vi "S4ACS_GUI.vi"() -> ()   [LabVIEW 2012]
uses:
  StateMachine/State Machine.lvclass
  Interface/Interface.lvclass
  S4ACS_GUI/S4ACS_GUI.lvclass
  Channel/Channel.lvclass
  Acquisition/Acquisition.lvclass
  Trigger/Trigger.lvclass
  SyncBox/Sync Box.lvclass
panel:
  in  "SyncBox Setup":enum32{"Page 1"}(tab)
  in  "Set SyncBox":bool
  in  "DelayA":string
  in  "DelayB":string
  in  "DelayC":string
  in  "DelayD":string
  in  "SyncBox":bool
  in  "DS9":bool
  in  "Comments":string
  in  "Observation Title":string
  in  "Image Path":path
  in  "File Basename":string
  in  "# Index":u32
  in  "# Images":u32
  out "error out":errorcluster
  in  "Kinetic Series Length":u8=1 min=1 max=80
  in  "Final Line":u16=1024 min=1 max=1024
  in  "Image Name":string="CH1"
  in  "Final Column":u16=1024 min=1 max=1024
  in  "Initial Cloumn":u16=1 min=1 max=1024
  in  "# Ciclos":u32=1 min=1
  in  "Exposure Time":dbl=1e-05 min=1e-05
  in  "Initial Line":u16=1 min=1 max=1024
  in  "Binning 5":u8=1 min=1 max=2
  in  "EM Gain":u16=2 min=2 max=300
  in  "EM Mode":u8(ring) items=["Electron Multiplying", "Conventional"]
  in  "Pre-amp gain":u8(ring) items=["Gain 1", "Gain 2"]
  in  "Readout Rate":u8(ring) items=["30 MHz", "20 MHz", "10 MHz", "  1 MHz"]
  in  "Night Directory":string="C:\\Users\\observer\\Desktop\\SPARC4 Acquisition Control\\Imagens"
  in  "Camera Setup":T1={"Image Name"="Image", "Image Path"="C:\\Users\\Cliente\\Desktop\\SPARC4_AC\\Imagens\\", "# Images"=0, "Exposure Time"=0.0, "Pre-amp gain"=0, "Readout Rate"=0, "Vertical Shift Speed"=3, "Acquisition Mode"=1, "Read Mode"=4, "EM Mode"=0, "EM Gain"=2, "Shutter Mode"=2, "Shutter TTL"=0, "Time to open shutter"=50, "Time to close shutter"=50, "Vertical Binning"=1, "Horizontal Binning"=1, "Initial Line"=1, "Initial Cloumn"=1, "Final Line"=1024, "Final Column"=1024, "Cooler ON/OFF"=0, "Set temperature"=20, "Number of exp"=0, "Exposições realizadas"=0, "Kinetic Serie Length"=0, "Number of Accumulations"=0, "Kinetic Cycle Time"=0, "Frame Transfer"=FALSE, "Vertical Clock Amplitude"=0, "Trigger"=0} {"Trigger" items=["Internal", "External", "N/A", "N/A", "N/A", "N/A", "External Start"]; "Vertical Clock Amplitude" items=["Normal", "+1", "+2", "+3", "+4"]; "Set temperature" min=0 max=0; "Cooler ON/OFF" items=["Cooler OFF", "Cooler ON"]; "Shutter TTL" items=["TTL Low", "TTl High"]; "Shutter Mode" items=["Fully Auto", "OPEN", "CLOSED"]; "EM Mode" items=["Electron Multiplying", "Conventional"]; "Read Mode" items=["Full Vertical Binning", "Multi-Track", "Random-track", "Single-Track", "Image"]; "Acquisition Mode" items=["N/A", "Single", "Accumulate", "Kinetic", "Fast Kinetic"]; "Vertical Shift Speed" items=["0.6", "1.13", "2.2", "4.33"]; "Readout Rate" items=["1 MHz", "10 MHz", "20 MHz", "30 MHz"]; "Pre-amp gain" items=["Gain 1", "Gain 2"]}
  in  "Adquirir":bool
  in  "Adquirir 3":bool
  in  "Adquirir 4":bool
  in  "Adquirir 2":bool
  in  "stop":bool
  in  "S4ACS_GUI.lvclass":refnum<class "S4ACS_GUI.lvclass">
  # "Channel 1"
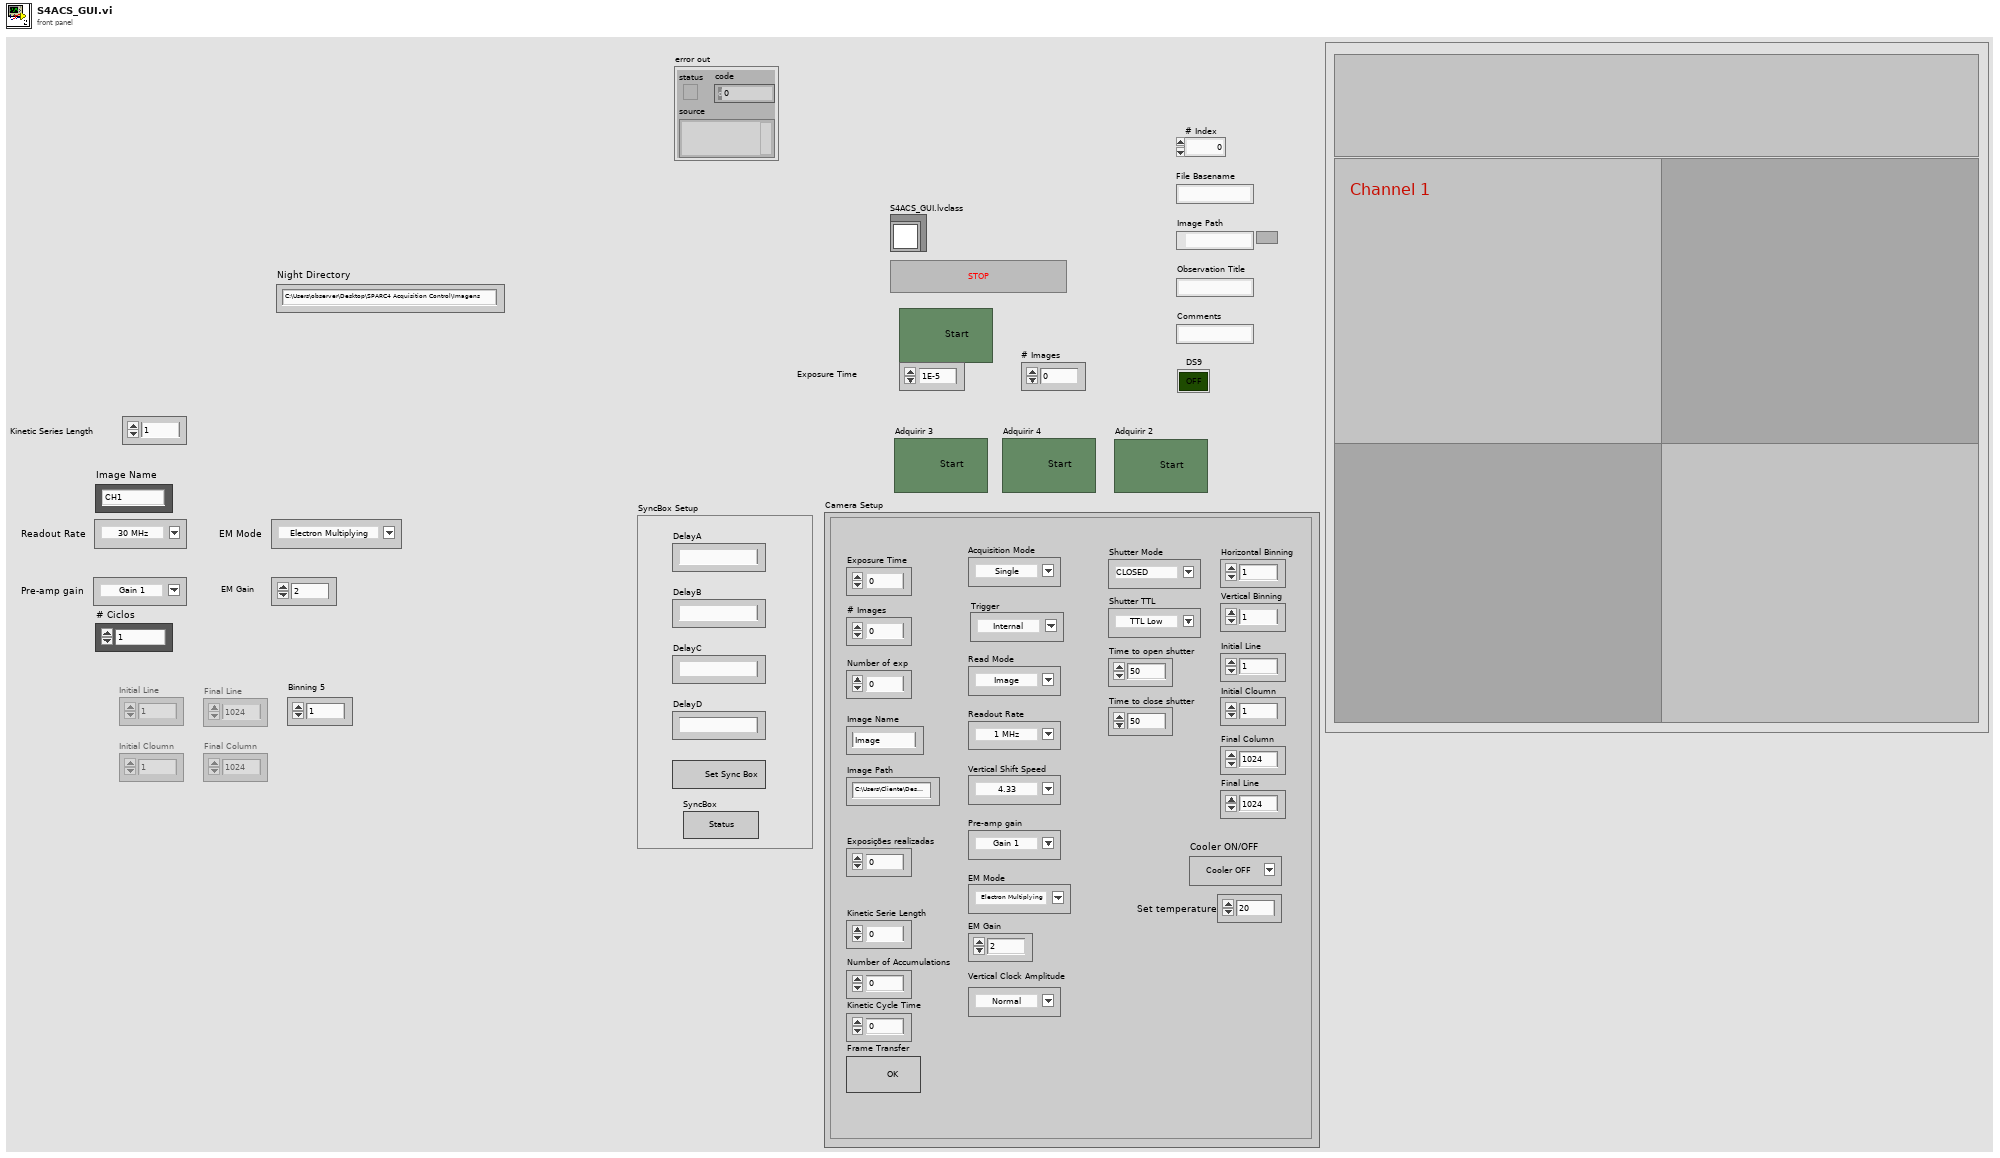
[diagram p1: front panel]
types:
  T1 = cluster{"Image Name":string, "Image Path":string, "# Images":u32, "Exposure Time":dbl, "Pre-amp gain":u8, "Readout Rate":u8, "Vertical Shift Speed":u8, "Acquisition Mode":u8, "Read Mode":u8, "EM Mode":u8, "EM Gain":u16, "Shutter Mode":u8, "Shutter TTL":u8, "Time to open shutter":u16, "Time to close shutter":u16, "Vertical Binning":u16, "Horizontal Binning":u16, "Initial Line":u16, "Initial Cloumn":u16, "Final Line":u16, "Final Column":u16, "Cooler ON/OFF":u16, "Set temperature":i8, "Number of exp":u32, "Exposições realizadas":u16, "Kinetic Serie Length":u32, "Number of Accumulations":u32, "Kinetic Cycle Time":u32, "Frame Transfer":bool, "Vertical Clock Amplitude":u8, "Trigger":u8}
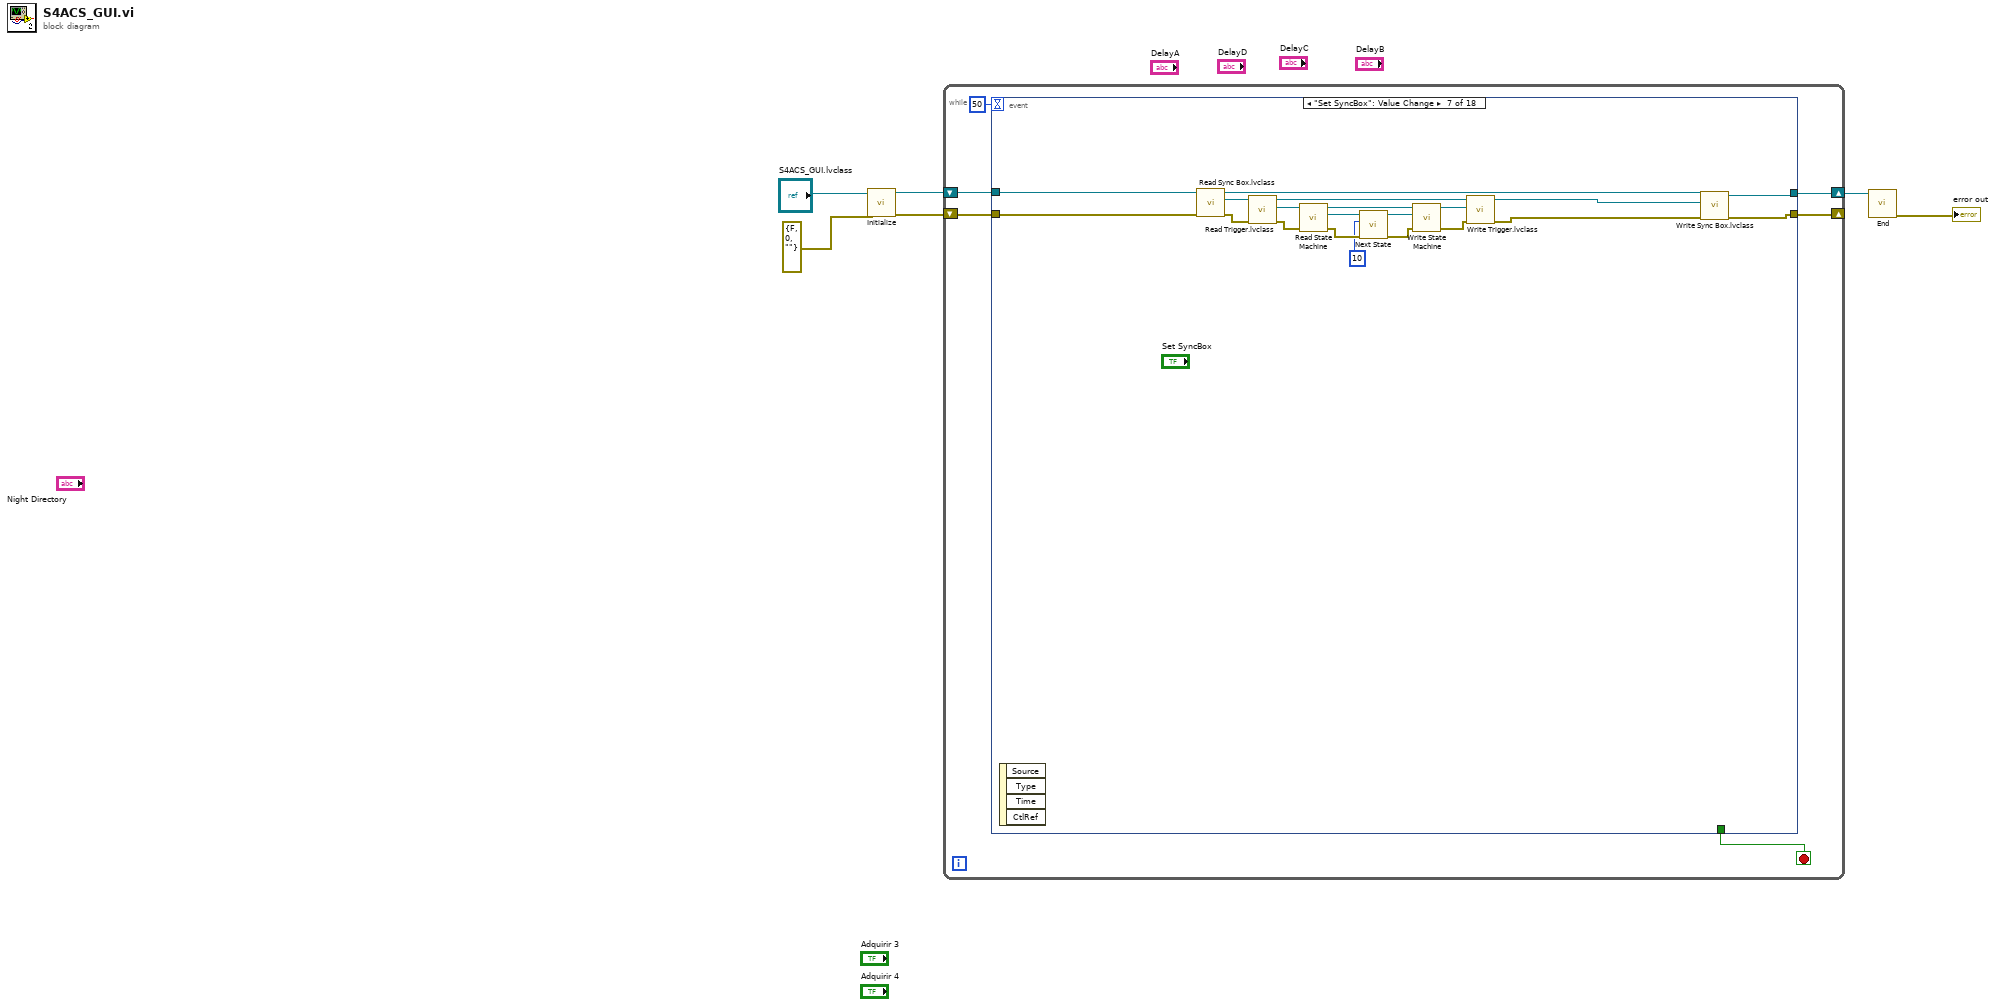
[diagram p0: block diagram]
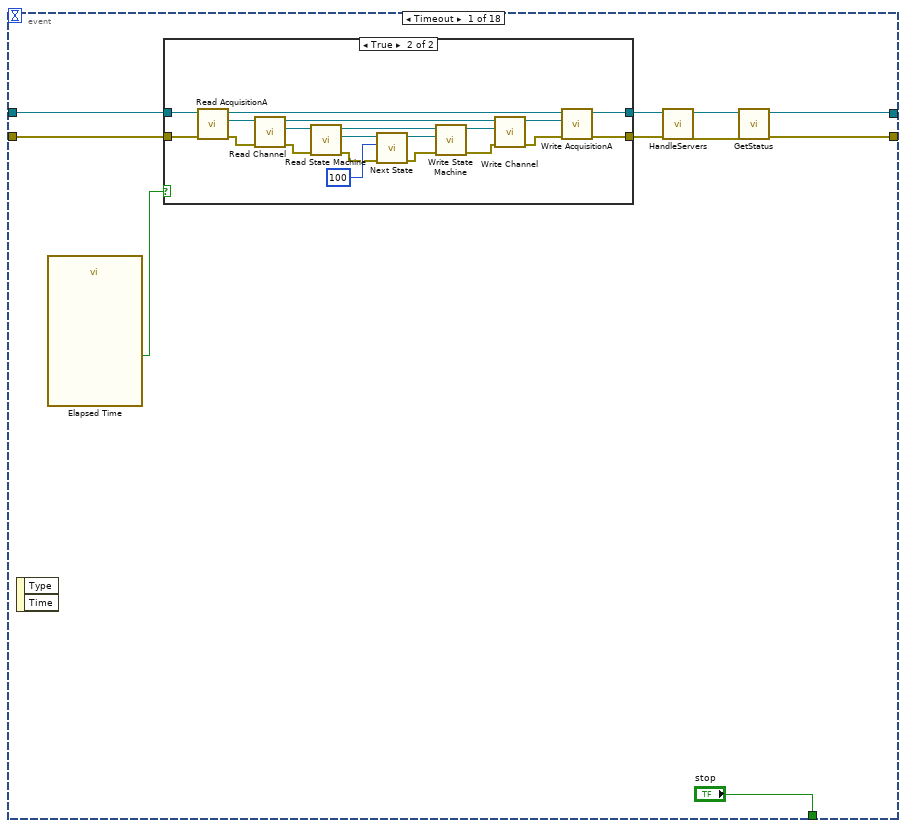
[diagram p2: hidden frame]
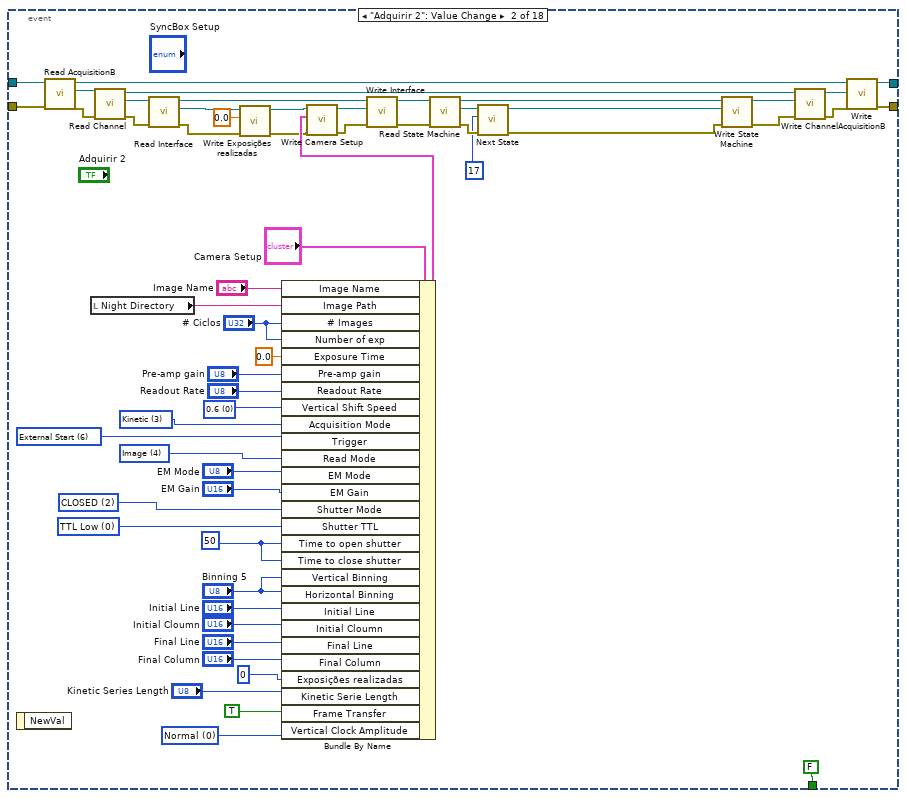
[diagram p4: hidden frame]
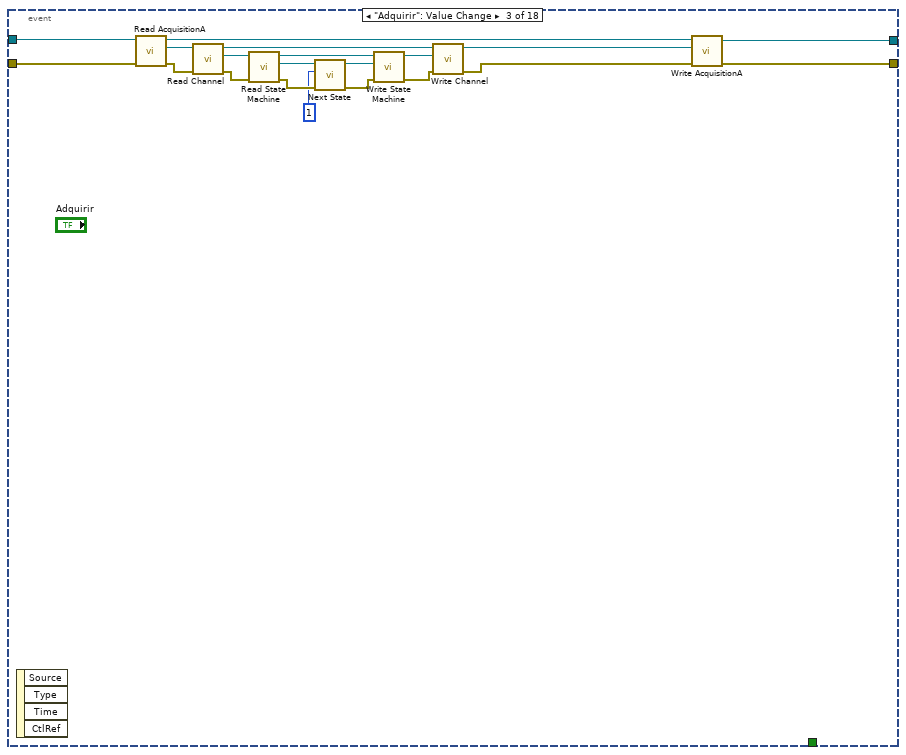
[diagram p5: hidden frame]
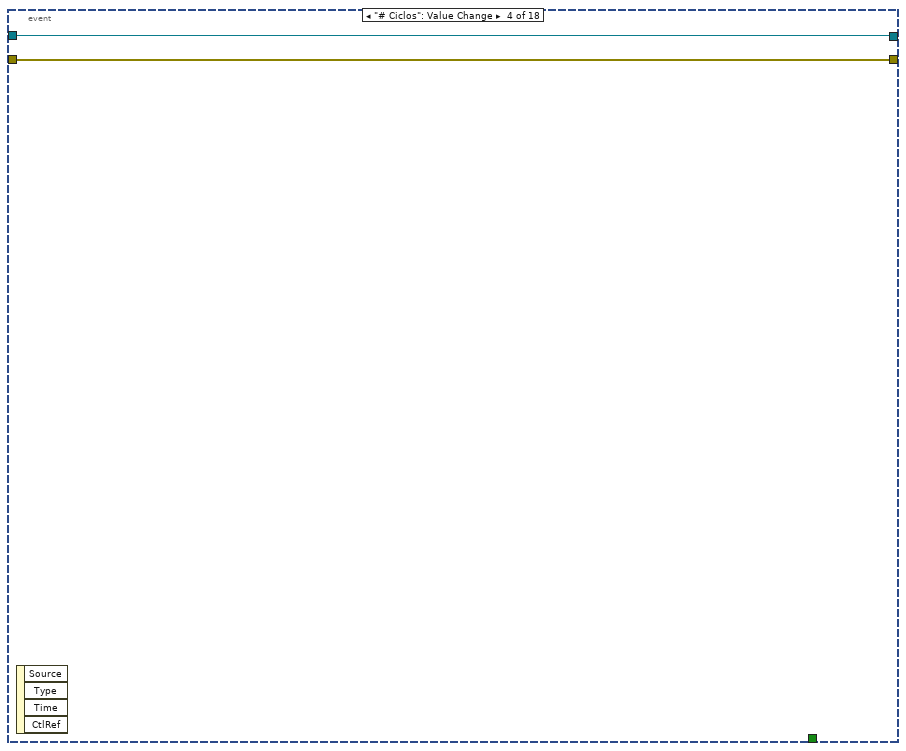
[diagram p6: hidden frame]
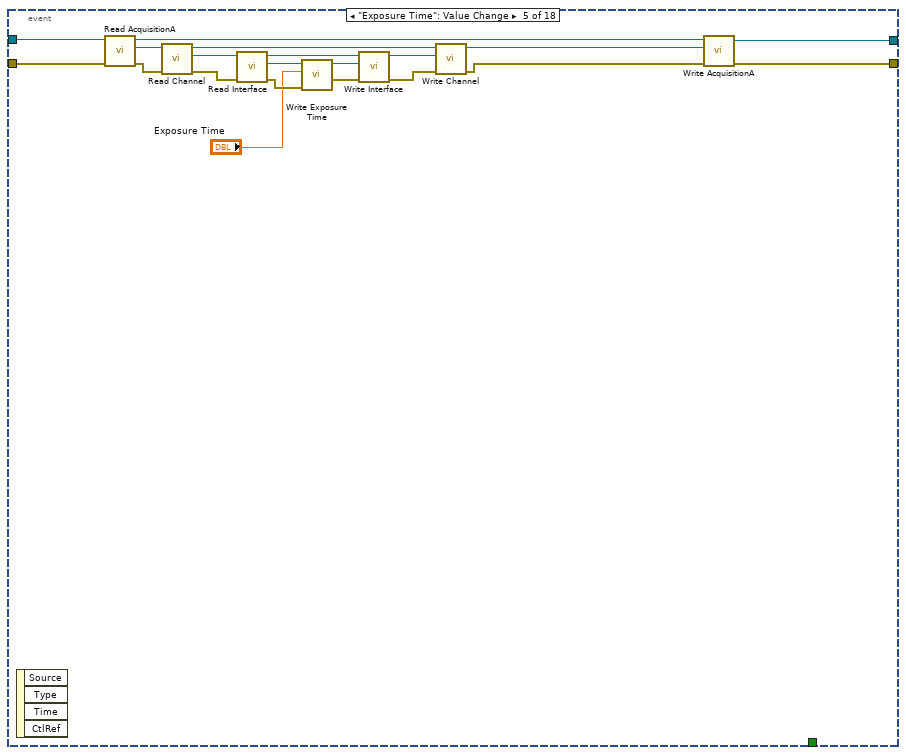
[diagram p7: hidden frame]
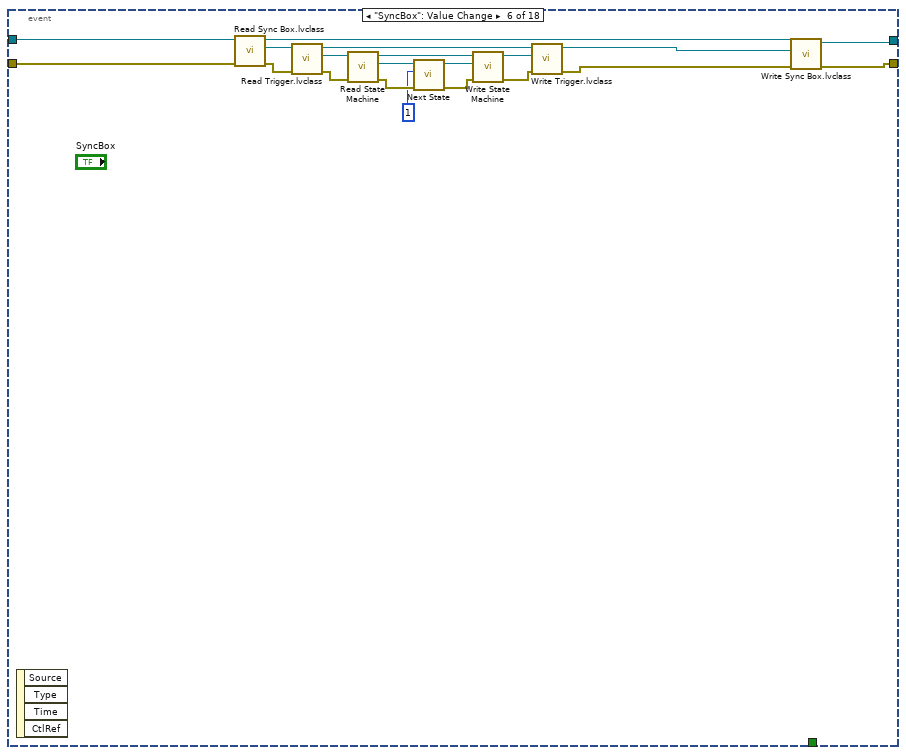
[diagram p8: hidden frame]
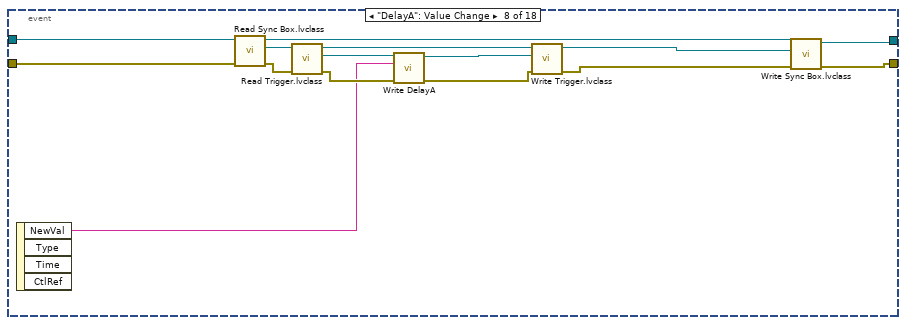
[diagram p9: hidden frame]
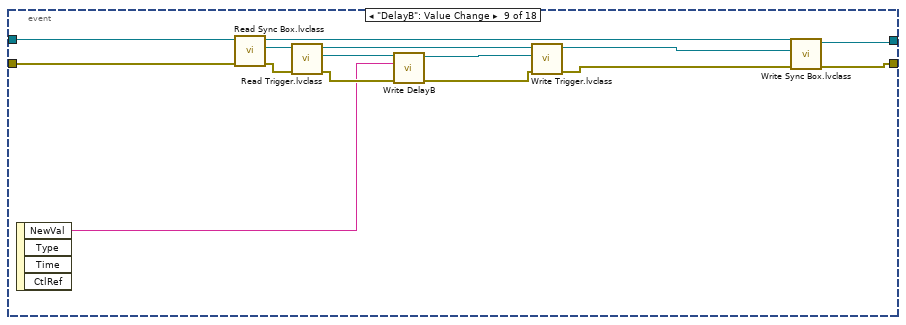
[diagram p10: hidden frame]
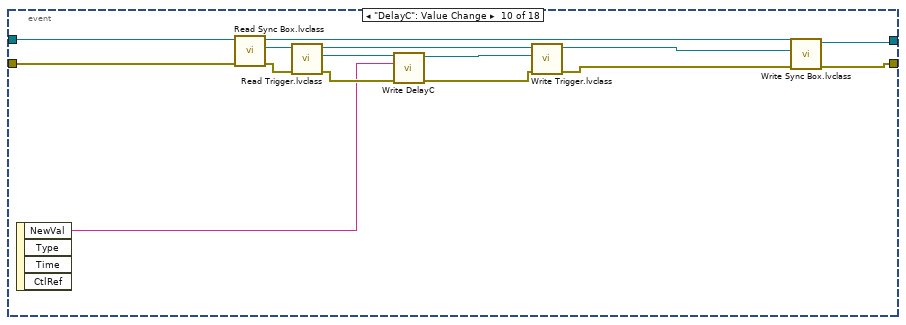
[diagram p11: hidden frame]
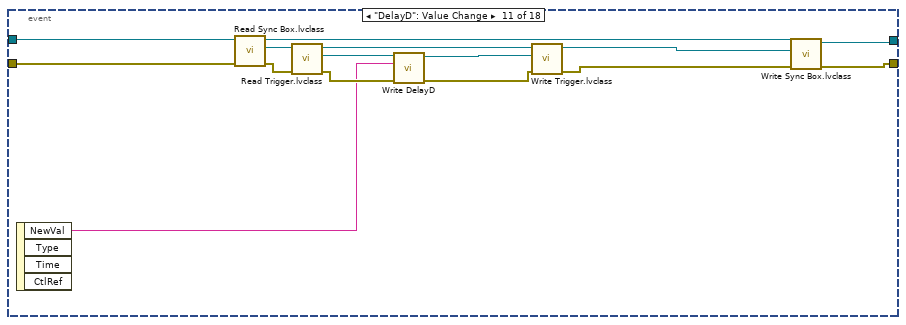
[diagram p12: hidden frame]
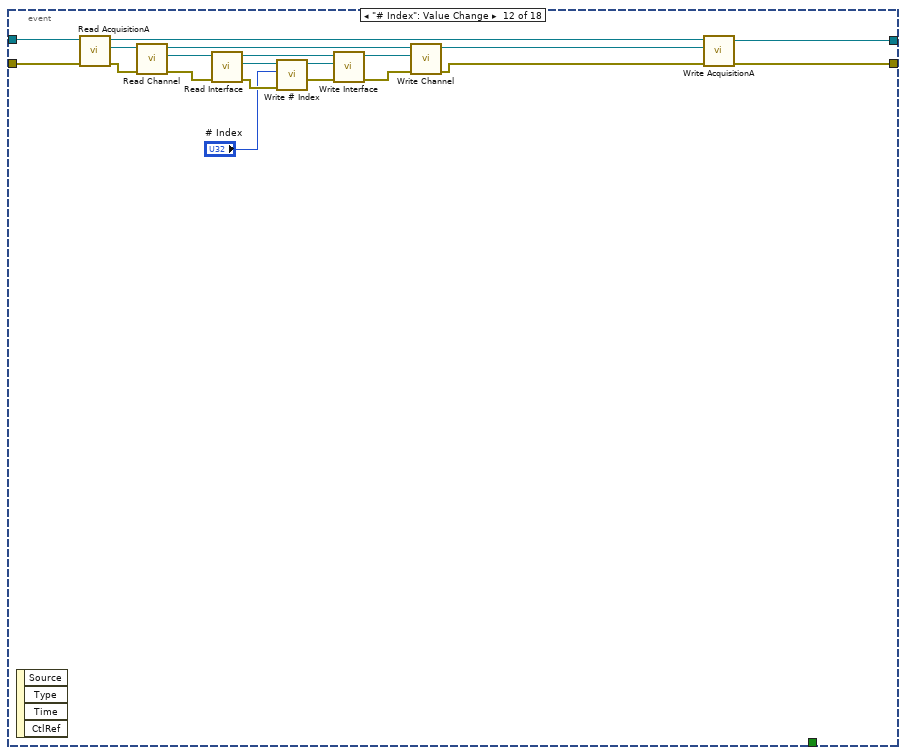
[diagram p13: hidden frame]
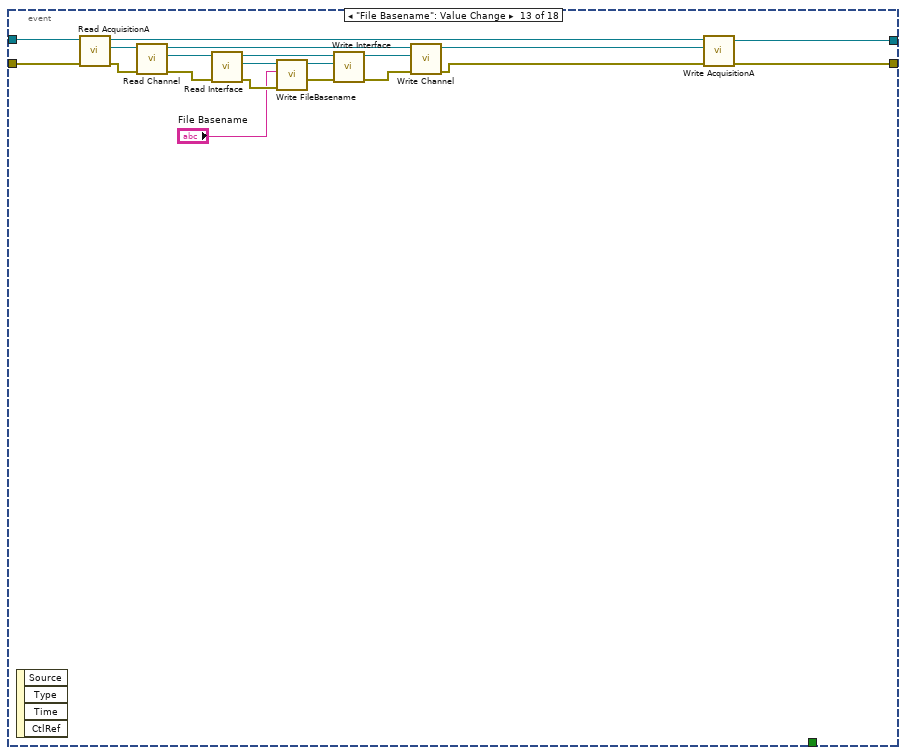
[diagram p14: hidden frame]
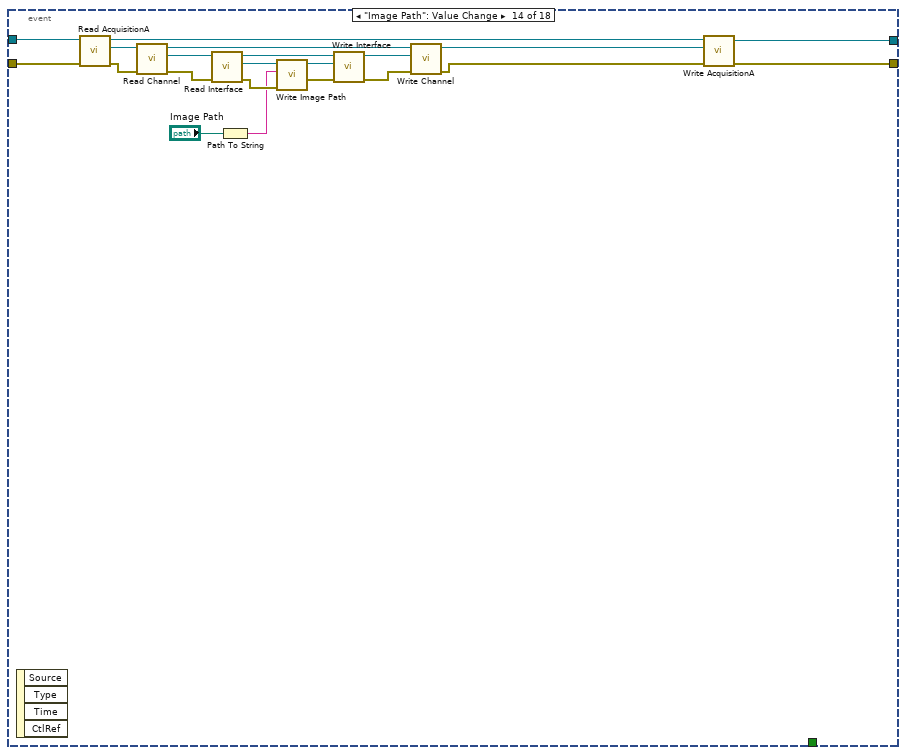
[diagram p15: hidden frame]
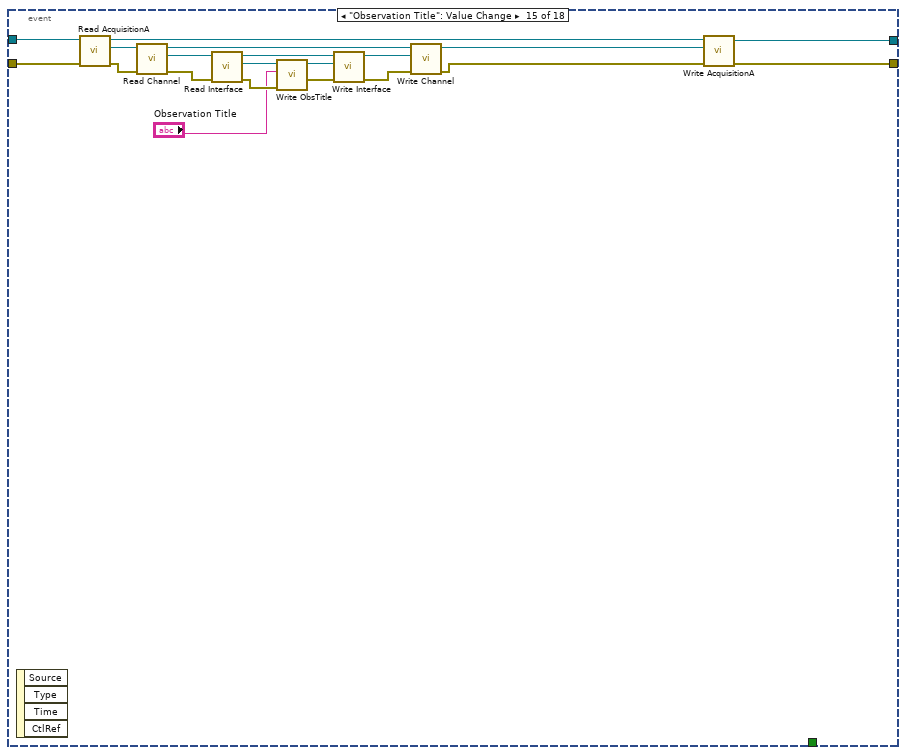
[diagram p16: hidden frame]
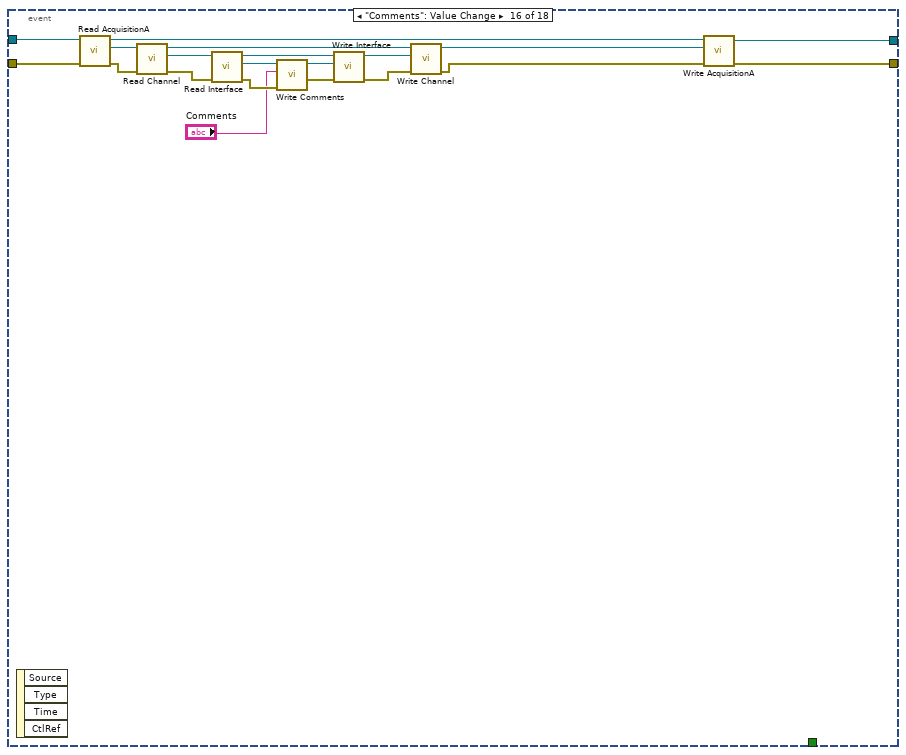
[diagram p17: hidden frame]
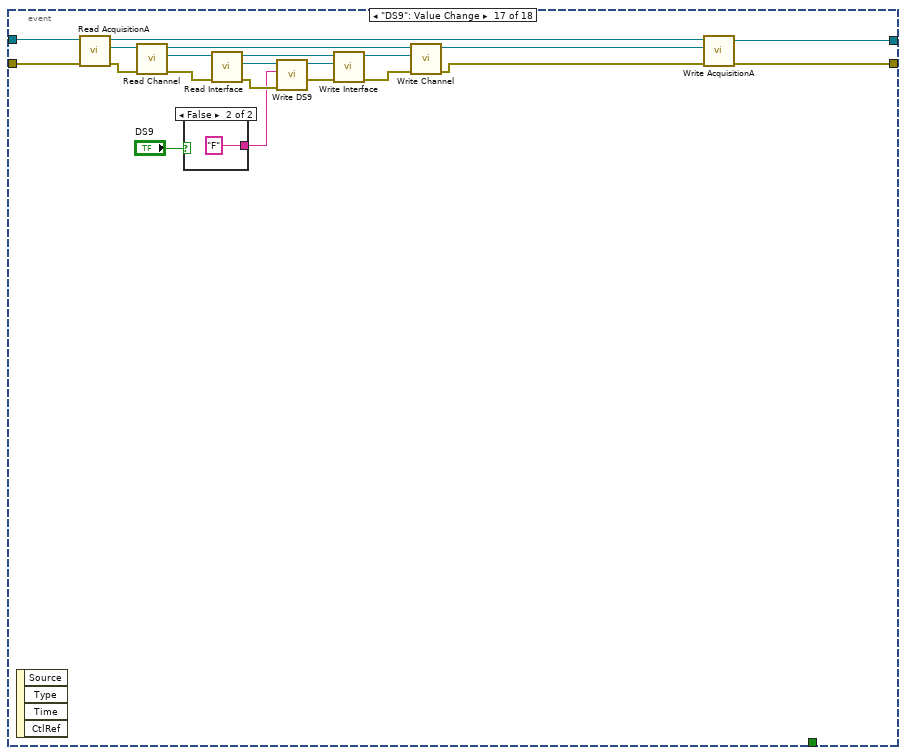
[diagram p18: hidden frame]
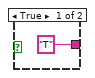
[diagram p19: hidden frame]
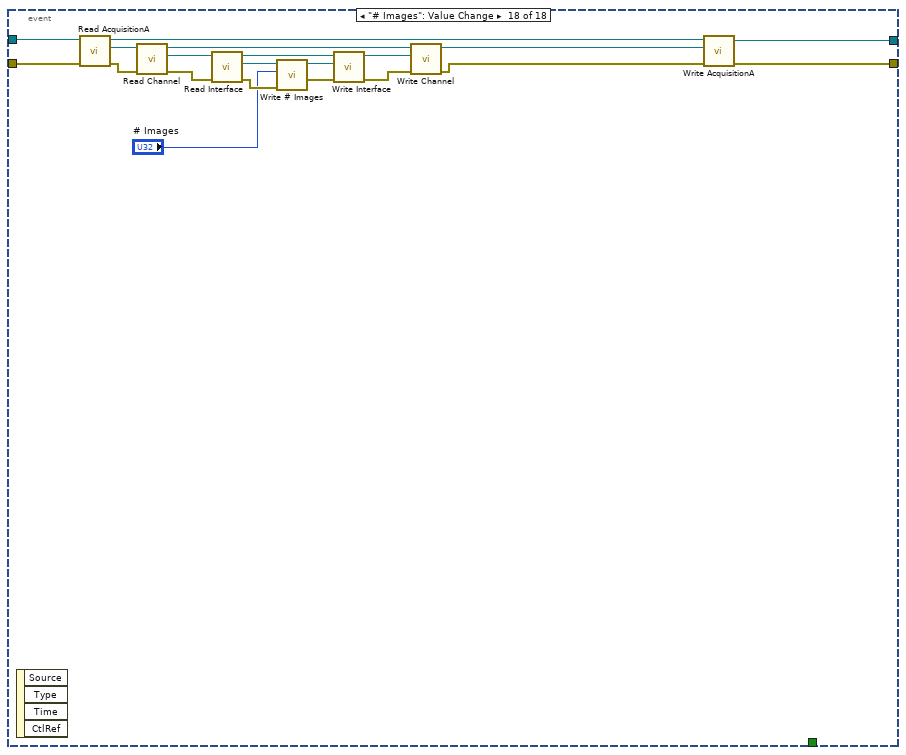
[diagram p20: hidden frame]
diagram:
  n1 = call-dynamic "Initialize.vi"("error in (no error)"=errorcluster {"status"=FALSE, "code"=0, "source"=""}, "S4ACS_GUI in"="S4ACS_GUI.lvclass") -> ("error out"=w3:errorcluster, "S4ACS_GUI out"=w4:refnum<class "S4ACS_GUI.lvclass">)  [unwired: 8 in]
  n2 = while {
    shift-right: [w10] -> w2
    shift-left: w4 -> [w12]
    shift-right: [w9] -> _
    shift-left: w3 -> [w11]
    stop <- w8 stop-if-true
    n3 = event shown="[6] \"Set SyncBox\": Value Change" {
      selector: _ -> [_ _ _ _ _ _ _ _ _ _ _ _ _ _ _ _ _ _]
      dyn-events: _ -> [_ _ _ _ _ _ _ _ _ _ _ _ _ _ _ _ _ _]
      timeout: 50 -> [_ _ _ _ _ _ _ _ _ _ _ _ _ _ _ _ _ _]
      tunnel: w12 -> [w17 w101 w121 w123 w143 w147 w167 w190 w205 w220 w235 w263 w283 w304 w324 w344 w365 w387]
      tunnel: w11 -> [w16 w78 w120 w122 w142 w146 w166 w189 w204 w219 w234 w262 w282 w303 w323 w343 w364 w386]
      tunnel: [w20 w71 w104 _ w134 w145 w165 w188 w203 w218 w233 w254 w274 w295 w315 w335 w356 w378] -> w9
      tunnel: [w19 w70 w105 w123 w135 w144 w164 w187 w202 w217 w232 w255 w275 w296 w316 w336 w357 w379] -> w10
      tunnel: ["stop" FALSE ("stop") _ _ _ _ _ _ _ _ _ _ _ _ _ _ _ _] -> w8
      tunnel: [_ _ _ w122 _ _ _ _ _ _ _ _ _ _ _ _ _ _] -> _
      event Timeout {
        n4 = event-data() -> ()  [unwired: 1 in, 2 out]
        n5 = call "Elapsed Time"() -> ("Time has Elapsed"=w13:bool)  [unwired: 12 in, 7 out]
        n6 = case shown="True" w13 {
          tunnel: w17 -> [w24 w31]
          tunnel: w16 -> [w23 w30]
          tunnel: [w24 w28] -> w15
          tunnel: [w23 w29] -> w14
          frame False {
          }
          frame True {
            n7 = call-dynamic "Read AcquisitionA.vi"("error in (no error)"=w30, "S4ACS_GUI in"=w31) -> ("error out"=w43:errorcluster, "Acquisition.lvclass"=w44:refnum<class "Acquisition.lvclass">, "S4ACS_GUI out"=w35:refnum<class "S4ACS_GUI.lvclass">)  [unwired: 7 in]
            n8 = call-dynamic "Read Channel.vi"("error in (no error)"=w43, "Acquisition in"=w44) -> ("error out"=w41:errorcluster, "Channel.lvclass"=w42:refnum<class "Channel.lvclass">, "Acquisition out"=w37:refnum<class "Acquisition.lvclass">)  [unwired: 7 in]
            n9 = call-dynamic "Read State Machine.vi"("error in (no error)"=w41, "Device in"=w42) -> ("error out"=w26:errorcluster, "State Machine.lvclass"=w40:refnum<class "State Machine.lvclass">, "Device out"=w38:refnum<class "Channel.lvclass">)  [unwired: 7 in]
            n10 = call "Next State.vi"("error in (no error)"=w26, "New_State"=u32 100, "State Machine in"=w40) -> ("error out"=w25:errorcluster, "State Machine out"=w39:refnum<class "State Machine.lvclass">)  [unwired: 7 in]
            n11 = call-dynamic "Write State Machine.vi"("error in (no error)"=w25, "State Machine.lvclass"=w39, "Device in"=w38) -> ("error out"=w33:errorcluster, "Device out"=w32:refnum<class "Channel.lvclass">)  [unwired: 7 in]
            n12 = call-dynamic "Write Channel.vi"("error in (no error)"=w33, "Channel.lvclass"=w32, "Acquisition in"=w37) -> ("error out"=w34:errorcluster, "Acquisition out"=w36:refnum<class "Acquisition.lvclass">)  [unwired: 7 in]
            n13 = call-dynamic "Write AcquisitionA.vi"("error in (no error)"=w34, "Acquisition.lvclass"=w36, "S4ACS_GUI in"=w35) -> ("error out"=w29:errorcluster, "S4ACS_GUI out"=w28:refnum<class "S4ACS_GUI.lvclass">)  [unwired: 7 in]
          }
        }
        n14 = call-dynamic "HandleServers.vi"("error in (no error)"=w14, "S4ACS_GUI in"=w15) -> ("error out"=w22:errorcluster, "S4ACS_GUI out"=w21:refnum<class "S4ACS_GUI.lvclass">)  [unwired: 8 in]
        n15 = call-dynamic "GetStatus.vi"("error in (no error)"=w22, "S4ACS_GUI in"=w21) -> ("error out"=w20:errorcluster, "S4ACS_GUI out"=w19:refnum<class "S4ACS_GUI.lvclass">)  [unwired: 8 in]
      }
      event "Adquirir 2": Value Change {
        w47 = u8 0 items=["Normal", "+1", "+2", "+3", "+4"] ("Vertical Clock Amplitude")
        w61 = u8 4 items=["Full Vertical Binning", "Multi-Track", "Random-track", "Single-Track", "Image"] ("Read Mode")
        w63 = u8 3 items=["N/A", "Single", "Accumulate", "Kinetic", "Fast Kinetic"] ("Acquisition Mode")
        w62 = u8 6 items=["Internal", "External", "RESERVED", "RESERVED", "RESERVED", "RESERVED", "External Start"] ("Trigger")
        w58 = u8 2 items=["Fully Auto", "OPEN", "CLOSED"] ("Shutter Mode")
        w57 = u8 0 items=["TTL Low", "TTl High"] ("Shutter TTL")
        w56 = u16 50 ("Time to open shutter")
        w64 = u8 0 items=["0.6", "1.13", "2.2", "4.33"] ("Vertical Shift Speed")
        n16 = event-data() -> ()  [unwired: 1 in, 1 out]
        n17 = call "Read AcquisitionB.vi"("error in (no error)"=w78, "S4ACS_GUI in"=w101) -> ("error out"=w77:errorcluster, "Acquisition.lvclass"=w100:refnum<class "Acquisition.lvclass">, "S4ACS_GUI out"=w88:refnum<class "S4ACS_GUI.lvclass">)  [unwired: 7 in]
        n18 = local read "Night Directory"() -> (w67:string)
        n19 = call-dynamic "Read Channel.vi"("error in (no error)"=w77, "Acquisition in"=w100) -> ("error out"=w76:errorcluster, "Channel.lvclass"=w99:refnum<class "Channel.lvclass">, "Acquisition out"=w86:refnum<class "Acquisition.lvclass">)  [unwired: 7 in]
        n20 = call-dynamic "Read Interface.vi"("error in (no error)"=w76, "Channel in"=w99) -> ("error out"=w75:errorcluster, "Interface.lvclass"=w98:refnum<class "Interface.lvclass">, "Channel out"=w93:refnum<class "Channel.lvclass">)  [unwired: 7 in]
        n21 = call-dynamic "Write Exposições realizadas.vi"("error in (no error)"=w75, "Exposições realizadas"=0.0, "Interface in"=w98) -> ("error out"=w74:errorcluster, "Interface out"=w97:refnum<class "Interface.lvclass">)  [unwired: 7 in]
        n22 = Bundle By Name(cluster="Camera Setup", "Image Name"="Image Name", "Image Path"=w67, "# Images"="# Ciclos", "Number of exp"="# Ciclos", "Exposure Time"=0.0, "Pre-amp gain"="Pre-amp gain", "Readout Rate"="Readout Rate", "Vertical Shift Speed"=w64, "Acquisition Mode"=w63, "Trigger"=w62, "Read Mode"=w61, "EM Mode"="EM Mode", "EM Gain"="EM Gain", "Shutter Mode"=w58, "Shutter TTL"=w57, "Time to open shutter"=w56, "Time to close shutter"=w56, "Vertical Binning"="Binning 5", "Horizontal Binning"="Binning 5", "Initial Line"="Initial Line", "Initial Cloumn"="Initial Cloumn", "Final Line"="Final Line", "Final Column"="Final Column", "Exposições realizadas"=u8 0, "Kinetic Serie Length"="Kinetic Series Length", "Frame Transfer"=TRUE, "Vertical Clock Amplitude"=w47) -> (w96:T1)
        n23 = call "Write Camera Setup.vi"("error in (no error)"=w74, "Camera Setup"=w96, "Interface in"=w97) -> ("error out"=w72:errorcluster, "Interface out"=w94:refnum<class "Interface.lvclass">)  [unwired: 7 in]
        n24 = call-dynamic "Write Interface.vi"("error in (no error)"=w72, "Interface.lvclass"=w94, "Channel in"=w93) -> ("error out"=w84:errorcluster, "Channel out"=w92:refnum<class "Channel.lvclass">)  [unwired: 7 in]
        n25 = call-dynamic "Read State Machine.vi"("error in (no error)"=w84, "Device in"=w92) -> ("error out"=w83:errorcluster, "State Machine.lvclass"=w91:refnum<class "State Machine.lvclass">, "Device out"=w89:refnum<class "Channel.lvclass">)  [unwired: 7 in]
        n26 = call "Next State.vi"("error in (no error)"=w83, "New_State"=u32 17, "State Machine in"=w91) -> ("error out"=w82:errorcluster, "State Machine out"=w90:refnum<class "State Machine.lvclass">)  [unwired: 7 in]
        n27 = call-dynamic "Write State Machine.vi"("error in (no error)"=w82, "State Machine.lvclass"=w90, "Device in"=w89) -> ("error out"=w81:errorcluster, "Device out"=w87:refnum<class "Channel.lvclass">)  [unwired: 7 in]
        n28 = call-dynamic "Write Channel.vi"("error in (no error)"=w81, "Channel.lvclass"=w87, "Acquisition in"=w86) -> ("error out"=w80:errorcluster, "Acquisition out"=w85:refnum<class "Acquisition.lvclass">)  [unwired: 7 in]
        n29 = call "Write AcquisitionB.vi"("error in (no error)"=w80, "Acquisition.lvclass"=w85, "S4ACS_GUI in"=w88) -> ("error out"=w71:errorcluster, "S4ACS_GUI out"=w70:refnum<class "S4ACS_GUI.lvclass">)  [unwired: 7 in]
      }
      event "Adquirir": Value Change {
        n30 = event-data() -> ()  [unwired: 1 in, 4 out]
        n31 = call-dynamic "Read AcquisitionA.vi"("error in (no error)"=w120, "S4ACS_GUI in"=w121) -> ("error out"=w118:errorcluster, "Acquisition.lvclass"=w119:refnum<class "Acquisition.lvclass">, "S4ACS_GUI out"=w107:refnum<class "S4ACS_GUI.lvclass">)  [unwired: 7 in]
        n32 = call-dynamic "Read Channel.vi"("error in (no error)"=w118, "Acquisition in"=w119) -> ("error out"=w116:errorcluster, "Channel.lvclass"=w117:refnum<class "Channel.lvclass">, "Acquisition out"=w110:refnum<class "Acquisition.lvclass">)  [unwired: 7 in]
        n33 = call-dynamic "Read State Machine.vi"("error in (no error)"=w116, "Device in"=w117) -> ("error out"=w114:errorcluster, "State Machine.lvclass"=w115:refnum<class "State Machine.lvclass">, "Device out"=w111:refnum<class "Channel.lvclass">)  [unwired: 7 in]
        n34 = call "Next State.vi"("error in (no error)"=w114, "New_State"=u32 1, "State Machine in"=w115) -> ("error out"=w109:errorcluster, "State Machine out"=w112:refnum<class "State Machine.lvclass">)  [unwired: 7 in]
        n35 = call-dynamic "Write State Machine.vi"("error in (no error)"=w109, "State Machine.lvclass"=w112, "Device in"=w111) -> ("error out"=w103:errorcluster, "Device out"=w102:refnum<class "Channel.lvclass">)  [unwired: 7 in]
        n36 = call-dynamic "Write Channel.vi"("error in (no error)"=w103, "Channel.lvclass"=w102, "Acquisition in"=w110) -> ("error out"=w106:errorcluster, "Acquisition out"=w108:refnum<class "Acquisition.lvclass">)  [unwired: 7 in]
        n37 = call-dynamic "Write AcquisitionA.vi"("error in (no error)"=w106, "Acquisition.lvclass"=w108, "S4ACS_GUI in"=w107) -> ("error out"=w104:errorcluster, "S4ACS_GUI out"=w105:refnum<class "S4ACS_GUI.lvclass">)  [unwired: 7 in]
      }
      event "# Ciclos": Value Change {
        n38 = event-data() -> ()  [unwired: 1 in, 4 out]
      }
      event "Exposure Time": Value Change {
        n39 = event-data() -> ()  [unwired: 1 in, 4 out]
        n40 = call-dynamic "Read AcquisitionA.vi"("error in (no error)"=w142, "S4ACS_GUI in"=w143) -> ("error out"=w140:errorcluster, "Acquisition.lvclass"=w141:refnum<class "Acquisition.lvclass">, "S4ACS_GUI out"=w137:refnum<class "S4ACS_GUI.lvclass">)  [unwired: 7 in]
        n41 = call-dynamic "Read Channel.vi"("error in (no error)"=w140, "Acquisition in"=w141) -> ("error out"=w125:errorcluster, "Channel.lvclass"=w126:refnum<class "Channel.lvclass">, "Acquisition out"=w139:refnum<class "Acquisition.lvclass">)  [unwired: 7 in]
        n42 = call-dynamic "Read Interface.vi"("error in (no error)"=w125, "Channel in"=w126) -> ("error out"=w132:errorcluster, "Interface.lvclass"=w133:refnum<class "Interface.lvclass">, "Channel out"=w130:refnum<class "Channel.lvclass">)  [unwired: 7 in]
        n43 = call "Write Exposure Time.vi"("error in (no error)"=w132, "Exposure Time"="Exposure Time", "Interface in"=w133) -> ("error out"=w127:errorcluster, "Interface out"=w131:refnum<class "Interface.lvclass">)  [unwired: 7 in]
        n44 = call-dynamic "Write Interface.vi"("error in (no error)"=w127, "Interface.lvclass"=w131, "Channel in"=w130) -> ("error out"=w128:errorcluster, "Channel out"=w129:refnum<class "Channel.lvclass">)  [unwired: 7 in]
        n45 = call-dynamic "Write Channel.vi"("error in (no error)"=w128, "Channel.lvclass"=w129, "Acquisition in"=w139) -> ("error out"=w136:errorcluster, "Acquisition out"=w138:refnum<class "Acquisition.lvclass">)  [unwired: 7 in]
        n46 = call-dynamic "Write AcquisitionA.vi"("error in (no error)"=w136, "Acquisition.lvclass"=w138, "S4ACS_GUI in"=w137) -> ("error out"=w134:errorcluster, "S4ACS_GUI out"=w135:refnum<class "S4ACS_GUI.lvclass">)  [unwired: 7 in]
      }
      event "SyncBox": Value Change {
        n47 = event-data() -> ()  [unwired: 1 in, 4 out]
        n48 = call-dynamic "Read Sync Box.lvclass.vi"("error in (no error)"=w146, "SPARC4_AC in"=w147) -> ("error out"=w162:errorcluster, "Sync Box.lvclass"=w163:refnum<class "Sync Box.lvclass">, "SPARC4_AC out"=w151:refnum<class "S4ACS_GUI.lvclass">)  [unwired: 7 in]
        n49 = call-dynamic "Read Trigger.lvclass.vi"("error in (no error)"=w162, "Sync Box in"=w163) -> ("error out"=w160:errorcluster, "Trigger.lvclass"=w161:refnum<class "Trigger.lvclass">, "Sync Box out"=w154:refnum<class "Sync Box.lvclass">)  [unwired: 7 in]
        n50 = call-dynamic "Read State Machine.vi"("error in (no error)"=w160, "Device in"=w161) -> ("error out"=w158:errorcluster, "State Machine.lvclass"=w159:refnum<class "State Machine.lvclass">, "Device out"=w155:refnum<class "Trigger.lvclass">)  [unwired: 7 in]
        n51 = call "Next State.vi"("error in (no error)"=w158, "New_State"=u32 1, "State Machine in"=w159) -> ("error out"=w153:errorcluster, "State Machine out"=w156:refnum<class "State Machine.lvclass">)  [unwired: 7 in]
        n52 = call-dynamic "Write State Machine.vi"("error in (no error)"=w153, "State Machine.lvclass"=w156, "Device in"=w155) -> ("error out"=w149:errorcluster, "Device out"=w148:refnum<class "Trigger.lvclass">)  [unwired: 7 in]
        n53 = call-dynamic "Write Trigger.lvclass.vi"("error in (no error)"=w149, "Trigger.lvclass"=w148, "Sync Box in"=w154) -> ("error out"=w150:errorcluster, "Sync Box out"=w152:refnum<class "Sync Box.lvclass">)  [unwired: 7 in]
        n54 = call-dynamic "Write Sync Box.lvclass.vi"("error in (no error)"=w150, "Sync Box.lvclass"=w152, "SPARC4_AC in"=w151) -> ("error out"=w145:errorcluster, "SPARC4_AC out"=w144:refnum<class "S4ACS_GUI.lvclass">)  [unwired: 7 in]
      }
      event "Set SyncBox": Value Change {
        n55 = event-data() -> ()  [unwired: 1 in, 4 out]
        n56 = call-dynamic "Read Sync Box.lvclass.vi"("error in (no error)"=w166, "SPARC4_AC in"=w167) -> ("error out"=w182:errorcluster, "Sync Box.lvclass"=w183:refnum<class "Sync Box.lvclass">, "SPARC4_AC out"=w171:refnum<class "S4ACS_GUI.lvclass">)  [unwired: 7 in]
        n57 = call-dynamic "Read Trigger.lvclass.vi"("error in (no error)"=w182, "Sync Box in"=w183) -> ("error out"=w180:errorcluster, "Trigger.lvclass"=w181:refnum<class "Trigger.lvclass">, "Sync Box out"=w174:refnum<class "Sync Box.lvclass">)  [unwired: 7 in]
        n58 = call-dynamic "Read State Machine.vi"("error in (no error)"=w180, "Device in"=w181) -> ("error out"=w178:errorcluster, "State Machine.lvclass"=w179:refnum<class "State Machine.lvclass">, "Device out"=w175:refnum<class "Trigger.lvclass">)  [unwired: 7 in]
        n59 = call "Next State.vi"("error in (no error)"=w178, "New_State"=u32 10, "State Machine in"=w179) -> ("error out"=w173:errorcluster, "State Machine out"=w176:refnum<class "State Machine.lvclass">)  [unwired: 7 in]
        n60 = call-dynamic "Write State Machine.vi"("error in (no error)"=w173, "State Machine.lvclass"=w176, "Device in"=w175) -> ("error out"=w169:errorcluster, "Device out"=w168:refnum<class "Trigger.lvclass">)  [unwired: 7 in]
        n61 = call-dynamic "Write Trigger.lvclass.vi"("error in (no error)"=w169, "Trigger.lvclass"=w168, "Sync Box in"=w174) -> ("error out"=w170:errorcluster, "Sync Box out"=w172:refnum<class "Sync Box.lvclass">)  [unwired: 7 in]
        n62 = call-dynamic "Write Sync Box.lvclass.vi"("error in (no error)"=w170, "Sync Box.lvclass"=w172, "SPARC4_AC in"=w171) -> ("error out"=w165:errorcluster, "SPARC4_AC out"=w164:refnum<class "S4ACS_GUI.lvclass">)  [unwired: 7 in]
      }
      event "DelayA": Value Change {
        n63 = event-data() -> ("NewVal"=w184:string)  [unwired: 1 in, 3 out]
        n64 = call-dynamic "Read Sync Box.lvclass.vi"("error in (no error)"=w189, "SPARC4_AC in"=w190) -> ("error out"=w197:errorcluster, "Sync Box.lvclass"=w198:refnum<class "Sync Box.lvclass">, "SPARC4_AC out"=w194:refnum<class "S4ACS_GUI.lvclass">)  [unwired: 7 in]
        n65 = call-dynamic "Read Trigger.lvclass.vi"("error in (no error)"=w197, "Sync Box in"=w198) -> ("error out"=w185:errorcluster, "Trigger.lvclass"=w186:refnum<class "Trigger.lvclass">, "Sync Box out"=w196:refnum<class "Sync Box.lvclass">)  [unwired: 7 in]
        n66 = call-dynamic "Write DelayA.vi"("error in (no error)"=w185, "DelayA"=w184, "Trigger in"=w186) -> ("error out"=w192:errorcluster, "Trigger out"=w191:refnum<class "Trigger.lvclass">)  [unwired: 7 in]
        n67 = call-dynamic "Write Trigger.lvclass.vi"("error in (no error)"=w192, "Trigger.lvclass"=w191, "Sync Box in"=w196) -> ("error out"=w193:errorcluster, "Sync Box out"=w195:refnum<class "Sync Box.lvclass">)  [unwired: 7 in]
        n68 = call-dynamic "Write Sync Box.lvclass.vi"("error in (no error)"=w193, "Sync Box.lvclass"=w195, "SPARC4_AC in"=w194) -> ("error out"=w188:errorcluster, "SPARC4_AC out"=w187:refnum<class "S4ACS_GUI.lvclass">)  [unwired: 7 in]
      }
      event "DelayB": Value Change {
        n69 = event-data() -> ("NewVal"=w199:string)  [unwired: 1 in, 3 out]
        n70 = call-dynamic "Read Sync Box.lvclass.vi"("error in (no error)"=w204, "SPARC4_AC in"=w205) -> ("error out"=w212:errorcluster, "Sync Box.lvclass"=w213:refnum<class "Sync Box.lvclass">, "SPARC4_AC out"=w209:refnum<class "S4ACS_GUI.lvclass">)  [unwired: 7 in]
        n71 = call-dynamic "Read Trigger.lvclass.vi"("error in (no error)"=w212, "Sync Box in"=w213) -> ("error out"=w200:errorcluster, "Trigger.lvclass"=w201:refnum<class "Trigger.lvclass">, "Sync Box out"=w211:refnum<class "Sync Box.lvclass">)  [unwired: 7 in]
        n72 = call-dynamic "Write DelayB.vi"("error in (no error)"=w200, "DelayB"=w199, "Trigger in"=w201) -> ("error out"=w207:errorcluster, "Trigger out"=w206:refnum<class "Trigger.lvclass">)  [unwired: 7 in]
        n73 = call-dynamic "Write Trigger.lvclass.vi"("error in (no error)"=w207, "Trigger.lvclass"=w206, "Sync Box in"=w211) -> ("error out"=w208:errorcluster, "Sync Box out"=w210:refnum<class "Sync Box.lvclass">)  [unwired: 7 in]
        n74 = call-dynamic "Write Sync Box.lvclass.vi"("error in (no error)"=w208, "Sync Box.lvclass"=w210, "SPARC4_AC in"=w209) -> ("error out"=w203:errorcluster, "SPARC4_AC out"=w202:refnum<class "S4ACS_GUI.lvclass">)  [unwired: 7 in]
      }
      event "DelayC": Value Change {
        n75 = event-data() -> ("NewVal"=w214:string)  [unwired: 1 in, 3 out]
        n76 = call-dynamic "Read Sync Box.lvclass.vi"("error in (no error)"=w219, "SPARC4_AC in"=w220) -> ("error out"=w227:errorcluster, "Sync Box.lvclass"=w228:refnum<class "Sync Box.lvclass">, "SPARC4_AC out"=w224:refnum<class "S4ACS_GUI.lvclass">)  [unwired: 7 in]
        n77 = call-dynamic "Read Trigger.lvclass.vi"("error in (no error)"=w227, "Sync Box in"=w228) -> ("error out"=w215:errorcluster, "Trigger.lvclass"=w216:refnum<class "Trigger.lvclass">, "Sync Box out"=w226:refnum<class "Sync Box.lvclass">)  [unwired: 7 in]
        n78 = call-dynamic "Write DelayC.vi"("error in (no error)"=w215, "DelayC"=w214, "Trigger in"=w216) -> ("error out"=w222:errorcluster, "Trigger out"=w221:refnum<class "Trigger.lvclass">)  [unwired: 7 in]
        n79 = call-dynamic "Write Trigger.lvclass.vi"("error in (no error)"=w222, "Trigger.lvclass"=w221, "Sync Box in"=w226) -> ("error out"=w223:errorcluster, "Sync Box out"=w225:refnum<class "Sync Box.lvclass">)  [unwired: 7 in]
        n80 = call-dynamic "Write Sync Box.lvclass.vi"("error in (no error)"=w223, "Sync Box.lvclass"=w225, "SPARC4_AC in"=w224) -> ("error out"=w218:errorcluster, "SPARC4_AC out"=w217:refnum<class "S4ACS_GUI.lvclass">)  [unwired: 7 in]
      }
      event "DelayD": Value Change {
        n81 = event-data() -> ("NewVal"=w229:string)  [unwired: 1 in, 3 out]
        n82 = call-dynamic "Read Sync Box.lvclass.vi"("error in (no error)"=w234, "SPARC4_AC in"=w235) -> ("error out"=w242:errorcluster, "Sync Box.lvclass"=w243:refnum<class "Sync Box.lvclass">, "SPARC4_AC out"=w239:refnum<class "S4ACS_GUI.lvclass">)  [unwired: 7 in]
        n83 = call-dynamic "Read Trigger.lvclass.vi"("error in (no error)"=w242, "Sync Box in"=w243) -> ("error out"=w230:errorcluster, "Trigger.lvclass"=w231:refnum<class "Trigger.lvclass">, "Sync Box out"=w241:refnum<class "Sync Box.lvclass">)  [unwired: 7 in]
        n84 = call-dynamic "Write DelayD.vi"("error in (no error)"=w230, "DelayD"=w229, "Trigger in"=w231) -> ("error out"=w237:errorcluster, "Trigger out"=w236:refnum<class "Trigger.lvclass">)  [unwired: 7 in]
        n85 = call-dynamic "Write Trigger.lvclass.vi"("error in (no error)"=w237, "Trigger.lvclass"=w236, "Sync Box in"=w241) -> ("error out"=w238:errorcluster, "Sync Box out"=w240:refnum<class "Sync Box.lvclass">)  [unwired: 7 in]
        n86 = call-dynamic "Write Sync Box.lvclass.vi"("error in (no error)"=w238, "Sync Box.lvclass"=w240, "SPARC4_AC in"=w239) -> ("error out"=w233:errorcluster, "SPARC4_AC out"=w232:refnum<class "S4ACS_GUI.lvclass">)  [unwired: 7 in]
      }
      event "# Index": Value Change {
        n87 = event-data() -> ()  [unwired: 1 in, 4 out]
        n88 = call-dynamic "Read AcquisitionA.vi"("error in (no error)"=w262, "S4ACS_GUI in"=w263) -> ("error out"=w260:errorcluster, "Acquisition.lvclass"=w261:refnum<class "Acquisition.lvclass">, "S4ACS_GUI out"=w257:refnum<class "S4ACS_GUI.lvclass">)  [unwired: 7 in]
        n89 = call-dynamic "Read Channel.vi"("error in (no error)"=w260, "Acquisition in"=w261) -> ("error out"=w245:errorcluster, "Channel.lvclass"=w246:refnum<class "Channel.lvclass">, "Acquisition out"=w259:refnum<class "Acquisition.lvclass">)  [unwired: 7 in]
        n90 = call-dynamic "Read Interface.vi"("error in (no error)"=w245, "Channel in"=w246) -> ("error out"=w252:errorcluster, "Interface.lvclass"=w253:refnum<class "Interface.lvclass">, "Channel out"=w250:refnum<class "Channel.lvclass">)  [unwired: 7 in]
        n91 = call-dynamic "Write # Index.vi"("error in (no error)"=w252, "# Index"="# Index", "Interface in"=w253) -> ("error out"=w247:errorcluster, "Interface out"=w251:refnum<class "Interface.lvclass">)  [unwired: 7 in]
        n92 = call-dynamic "Write Interface.vi"("error in (no error)"=w247, "Interface.lvclass"=w251, "Channel in"=w250) -> ("error out"=w248:errorcluster, "Channel out"=w249:refnum<class "Channel.lvclass">)  [unwired: 7 in]
        n93 = call-dynamic "Write Channel.vi"("error in (no error)"=w248, "Channel.lvclass"=w249, "Acquisition in"=w259) -> ("error out"=w256:errorcluster, "Acquisition out"=w258:refnum<class "Acquisition.lvclass">)  [unwired: 7 in]
        n94 = call-dynamic "Write AcquisitionA.vi"("error in (no error)"=w256, "Acquisition.lvclass"=w258, "S4ACS_GUI in"=w257) -> ("error out"=w254:errorcluster, "S4ACS_GUI out"=w255:refnum<class "S4ACS_GUI.lvclass">)  [unwired: 7 in]
      }
      event "File Basename": Value Change {
        n95 = event-data() -> ()  [unwired: 1 in, 4 out]
        n96 = call-dynamic "Read AcquisitionA.vi"("error in (no error)"=w282, "S4ACS_GUI in"=w283) -> ("error out"=w280:errorcluster, "Acquisition.lvclass"=w281:refnum<class "Acquisition.lvclass">, "S4ACS_GUI out"=w277:refnum<class "S4ACS_GUI.lvclass">)  [unwired: 7 in]
        n97 = call-dynamic "Read Channel.vi"("error in (no error)"=w280, "Acquisition in"=w281) -> ("error out"=w265:errorcluster, "Channel.lvclass"=w266:refnum<class "Channel.lvclass">, "Acquisition out"=w279:refnum<class "Acquisition.lvclass">)  [unwired: 7 in]
        n98 = call-dynamic "Read Interface.vi"("error in (no error)"=w265, "Channel in"=w266) -> ("error out"=w272:errorcluster, "Interface.lvclass"=w273:refnum<class "Interface.lvclass">, "Channel out"=w270:refnum<class "Channel.lvclass">)  [unwired: 7 in]
        n99 = call-dynamic "Write FileBasename.vi"("error in (no error)"=w272, "FileBasename"="File Basename", "Interface in"=w273) -> ("error out"=w267:errorcluster, "Interface out"=w271:refnum<class "Interface.lvclass">)  [unwired: 7 in]
        n100 = call-dynamic "Write Interface.vi"("error in (no error)"=w267, "Interface.lvclass"=w271, "Channel in"=w270) -> ("error out"=w268:errorcluster, "Channel out"=w269:refnum<class "Channel.lvclass">)  [unwired: 7 in]
        n101 = call-dynamic "Write Channel.vi"("error in (no error)"=w268, "Channel.lvclass"=w269, "Acquisition in"=w279) -> ("error out"=w276:errorcluster, "Acquisition out"=w278:refnum<class "Acquisition.lvclass">)  [unwired: 7 in]
        n102 = call-dynamic "Write AcquisitionA.vi"("error in (no error)"=w276, "Acquisition.lvclass"=w278, "S4ACS_GUI in"=w277) -> ("error out"=w274:errorcluster, "S4ACS_GUI out"=w275:refnum<class "S4ACS_GUI.lvclass">)  [unwired: 7 in]
      }
      event "Image Path": Value Change {
        n103 = event-data() -> ()  [unwired: 1 in, 4 out]
        n104 = call-dynamic "Read AcquisitionA.vi"("error in (no error)"=w303, "S4ACS_GUI in"=w304) -> ("error out"=w301:errorcluster, "Acquisition.lvclass"=w302:refnum<class "Acquisition.lvclass">, "S4ACS_GUI out"=w298:refnum<class "S4ACS_GUI.lvclass">)  [unwired: 7 in]
        n105 = call-dynamic "Read Channel.vi"("error in (no error)"=w301, "Acquisition in"=w302) -> ("error out"=w286:errorcluster, "Channel.lvclass"=w287:refnum<class "Channel.lvclass">, "Acquisition out"=w300:refnum<class "Acquisition.lvclass">)  [unwired: 7 in]
        n106 = call-dynamic "Read Interface.vi"("error in (no error)"=w286, "Channel in"=w287) -> ("error out"=w293:errorcluster, "Interface.lvclass"=w294:refnum<class "Interface.lvclass">, "Channel out"=w291:refnum<class "Channel.lvclass">)  [unwired: 7 in]
        n107 = Path To String(path="Image Path") -> (string=w284:string)
        n108 = call-dynamic "Write Image Path.vi"("error in (no error)"=w293, "Image Path"=w284, "Interface in"=w294) -> ("error out"=w288:errorcluster, "Interface out"=w292:refnum<class "Interface.lvclass">)  [unwired: 7 in]
        n109 = call-dynamic "Write Interface.vi"("error in (no error)"=w288, "Interface.lvclass"=w292, "Channel in"=w291) -> ("error out"=w289:errorcluster, "Channel out"=w290:refnum<class "Channel.lvclass">)  [unwired: 7 in]
        n110 = call-dynamic "Write Channel.vi"("error in (no error)"=w289, "Channel.lvclass"=w290, "Acquisition in"=w300) -> ("error out"=w297:errorcluster, "Acquisition out"=w299:refnum<class "Acquisition.lvclass">)  [unwired: 7 in]
        n111 = call-dynamic "Write AcquisitionA.vi"("error in (no error)"=w297, "Acquisition.lvclass"=w299, "S4ACS_GUI in"=w298) -> ("error out"=w295:errorcluster, "S4ACS_GUI out"=w296:refnum<class "S4ACS_GUI.lvclass">)  [unwired: 7 in]
      }
      event "Observation Title": Value Change {
        n112 = event-data() -> ()  [unwired: 1 in, 4 out]
        n113 = call-dynamic "Read AcquisitionA.vi"("error in (no error)"=w323, "S4ACS_GUI in"=w324) -> ("error out"=w321:errorcluster, "Acquisition.lvclass"=w322:refnum<class "Acquisition.lvclass">, "S4ACS_GUI out"=w318:refnum<class "S4ACS_GUI.lvclass">)  [unwired: 7 in]
        n114 = call-dynamic "Read Channel.vi"("error in (no error)"=w321, "Acquisition in"=w322) -> ("error out"=w306:errorcluster, "Channel.lvclass"=w307:refnum<class "Channel.lvclass">, "Acquisition out"=w320:refnum<class "Acquisition.lvclass">)  [unwired: 7 in]
        n115 = call-dynamic "Read Interface.vi"("error in (no error)"=w306, "Channel in"=w307) -> ("error out"=w313:errorcluster, "Interface.lvclass"=w314:refnum<class "Interface.lvclass">, "Channel out"=w311:refnum<class "Channel.lvclass">)  [unwired: 7 in]
        n116 = call-dynamic "Write ObsTitle.vi"("error in (no error)"=w313, "ObsTitle"="Observation Title", "Interface in"=w314) -> ("error out"=w308:errorcluster, "Interface out"=w312:refnum<class "Interface.lvclass">)  [unwired: 7 in]
        n117 = call-dynamic "Write Interface.vi"("error in (no error)"=w308, "Interface.lvclass"=w312, "Channel in"=w311) -> ("error out"=w309:errorcluster, "Channel out"=w310:refnum<class "Channel.lvclass">)  [unwired: 7 in]
        n118 = call-dynamic "Write Channel.vi"("error in (no error)"=w309, "Channel.lvclass"=w310, "Acquisition in"=w320) -> ("error out"=w317:errorcluster, "Acquisition out"=w319:refnum<class "Acquisition.lvclass">)  [unwired: 7 in]
        n119 = call-dynamic "Write AcquisitionA.vi"("error in (no error)"=w317, "Acquisition.lvclass"=w319, "S4ACS_GUI in"=w318) -> ("error out"=w315:errorcluster, "S4ACS_GUI out"=w316:refnum<class "S4ACS_GUI.lvclass">)  [unwired: 7 in]
      }
      event "Comments": Value Change {
        n120 = event-data() -> ()  [unwired: 1 in, 4 out]
        n121 = call-dynamic "Read AcquisitionA.vi"("error in (no error)"=w343, "S4ACS_GUI in"=w344) -> ("error out"=w341:errorcluster, "Acquisition.lvclass"=w342:refnum<class "Acquisition.lvclass">, "S4ACS_GUI out"=w338:refnum<class "S4ACS_GUI.lvclass">)  [unwired: 7 in]
        n122 = call-dynamic "Read Channel.vi"("error in (no error)"=w341, "Acquisition in"=w342) -> ("error out"=w326:errorcluster, "Channel.lvclass"=w327:refnum<class "Channel.lvclass">, "Acquisition out"=w340:refnum<class "Acquisition.lvclass">)  [unwired: 7 in]
        n123 = call-dynamic "Read Interface.vi"("error in (no error)"=w326, "Channel in"=w327) -> ("error out"=w333:errorcluster, "Interface.lvclass"=w334:refnum<class "Interface.lvclass">, "Channel out"=w331:refnum<class "Channel.lvclass">)  [unwired: 7 in]
        n124 = call-dynamic "Write Comments.vi"("error in (no error)"=w333, "Comments"="Comments", "Interface in"=w334) -> ("error out"=w328:errorcluster, "Interface out"=w332:refnum<class "Interface.lvclass">)  [unwired: 7 in]
        n125 = call-dynamic "Write Interface.vi"("error in (no error)"=w328, "Interface.lvclass"=w332, "Channel in"=w331) -> ("error out"=w329:errorcluster, "Channel out"=w330:refnum<class "Channel.lvclass">)  [unwired: 7 in]
        n126 = call-dynamic "Write Channel.vi"("error in (no error)"=w329, "Channel.lvclass"=w330, "Acquisition in"=w340) -> ("error out"=w337:errorcluster, "Acquisition out"=w339:refnum<class "Acquisition.lvclass">)  [unwired: 7 in]
        n127 = call-dynamic "Write AcquisitionA.vi"("error in (no error)"=w337, "Acquisition.lvclass"=w339, "S4ACS_GUI in"=w338) -> ("error out"=w335:errorcluster, "S4ACS_GUI out"=w336:refnum<class "S4ACS_GUI.lvclass">)  [unwired: 7 in]
      }
      event "DS9": Value Change {
        n128 = event-data() -> ()  [unwired: 1 in, 4 out]
        n129 = call-dynamic "Read AcquisitionA.vi"("error in (no error)"=w364, "S4ACS_GUI in"=w365) -> ("error out"=w362:errorcluster, "Acquisition.lvclass"=w363:refnum<class "Acquisition.lvclass">, "S4ACS_GUI out"=w359:refnum<class "S4ACS_GUI.lvclass">)  [unwired: 7 in]
        n130 = call-dynamic "Read Channel.vi"("error in (no error)"=w362, "Acquisition in"=w363) -> ("error out"=w347:errorcluster, "Channel.lvclass"=w348:refnum<class "Channel.lvclass">, "Acquisition out"=w361:refnum<class "Acquisition.lvclass">)  [unwired: 7 in]
        n131 = case shown="False" "DS9" {
          tunnel: ["T" "F"] -> w345
          frame True {
          }
          frame False {
          }
        }
        n132 = call-dynamic "Read Interface.vi"("error in (no error)"=w347, "Channel in"=w348) -> ("error out"=w354:errorcluster, "Interface.lvclass"=w355:refnum<class "Interface.lvclass">, "Channel out"=w352:refnum<class "Channel.lvclass">)  [unwired: 7 in]
        n133 = call-dynamic "Write DS9.vi"("error in (no error)"=w354, "DS9"=w345, "Interface in"=w355) -> ("error out"=w349:errorcluster, "Interface out"=w353:refnum<class "Interface.lvclass">)  [unwired: 7 in]
        n134 = call-dynamic "Write Interface.vi"("error in (no error)"=w349, "Interface.lvclass"=w353, "Channel in"=w352) -> ("error out"=w350:errorcluster, "Channel out"=w351:refnum<class "Channel.lvclass">)  [unwired: 7 in]
        n135 = call-dynamic "Write Channel.vi"("error in (no error)"=w350, "Channel.lvclass"=w351, "Acquisition in"=w361) -> ("error out"=w358:errorcluster, "Acquisition out"=w360:refnum<class "Acquisition.lvclass">)  [unwired: 7 in]
        n136 = call-dynamic "Write AcquisitionA.vi"("error in (no error)"=w358, "Acquisition.lvclass"=w360, "S4ACS_GUI in"=w359) -> ("error out"=w356:errorcluster, "S4ACS_GUI out"=w357:refnum<class "S4ACS_GUI.lvclass">)  [unwired: 7 in]
      }
      event "# Images": Value Change {
        n137 = event-data() -> ()  [unwired: 1 in, 4 out]
        n138 = call-dynamic "Read AcquisitionA.vi"("error in (no error)"=w386, "S4ACS_GUI in"=w387) -> ("error out"=w384:errorcluster, "Acquisition.lvclass"=w385:refnum<class "Acquisition.lvclass">, "S4ACS_GUI out"=w381:refnum<class "S4ACS_GUI.lvclass">)  [unwired: 7 in]
        n139 = call-dynamic "Read Channel.vi"("error in (no error)"=w384, "Acquisition in"=w385) -> ("error out"=w369:errorcluster, "Channel.lvclass"=w370:refnum<class "Channel.lvclass">, "Acquisition out"=w383:refnum<class "Acquisition.lvclass">)  [unwired: 7 in]
        n140 = call-dynamic "Read Interface.vi"("error in (no error)"=w369, "Channel in"=w370) -> ("error out"=w376:errorcluster, "Interface.lvclass"=w377:refnum<class "Interface.lvclass">, "Channel out"=w374:refnum<class "Channel.lvclass">)  [unwired: 7 in]
        n141 = call-dynamic "Write # Images.vi"("error in (no error)"=w376, "# Images"="# Images", "Interface in"=w377) -> ("error out"=w371:errorcluster, "Interface out"=w375:refnum<class "Interface.lvclass">)  [unwired: 7 in]
        n142 = call-dynamic "Write Interface.vi"("error in (no error)"=w371, "Interface.lvclass"=w375, "Channel in"=w374) -> ("error out"=w372:errorcluster, "Channel out"=w373:refnum<class "Channel.lvclass">)  [unwired: 7 in]
        n143 = call-dynamic "Write Channel.vi"("error in (no error)"=w372, "Channel.lvclass"=w373, "Acquisition in"=w383) -> ("error out"=w380:errorcluster, "Acquisition out"=w382:refnum<class "Acquisition.lvclass">)  [unwired: 7 in]
        n144 = call-dynamic "Write AcquisitionA.vi"("error in (no error)"=w380, "Acquisition.lvclass"=w382, "S4ACS_GUI in"=w381) -> ("error out"=w378:errorcluster, "S4ACS_GUI out"=w379:refnum<class "S4ACS_GUI.lvclass">)  [unwired: 7 in]
      }
    }
  }
  n145 = call-dynamic "End.vi"("S4ACS_GUI in"=w2) -> ("error out"=→"error out":errorcluster)  [unwired: 9 in, 1 out]
